vi "Calc RPM Vals.vi"(6 "RPM Loop Period (us)":u32, 10 "Sample Length(10)":u16, 11 "Inputs":bool[](array[boolean])=[FALSE, FALSE, FALSE, FALSE]) -> (3 "RPM Vals":sgl[](array[numeric]))   [LabVIEW 2018]
uses:
  <vilib>/rvi/Arithmetic/AddSubMult/XNode/nirviSatArithmetic.xnode
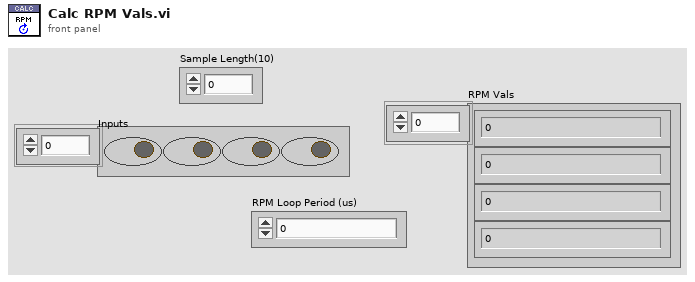
[diagram p1: front panel]
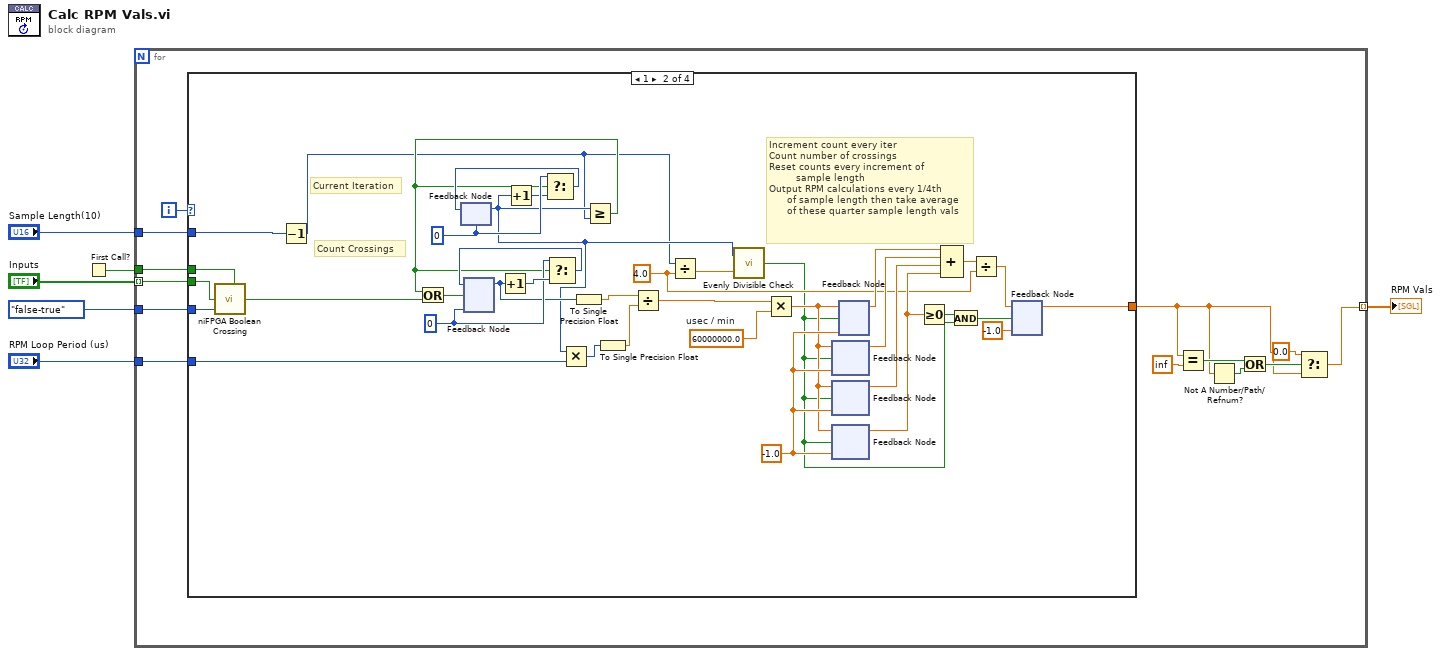
[diagram p0: block diagram]
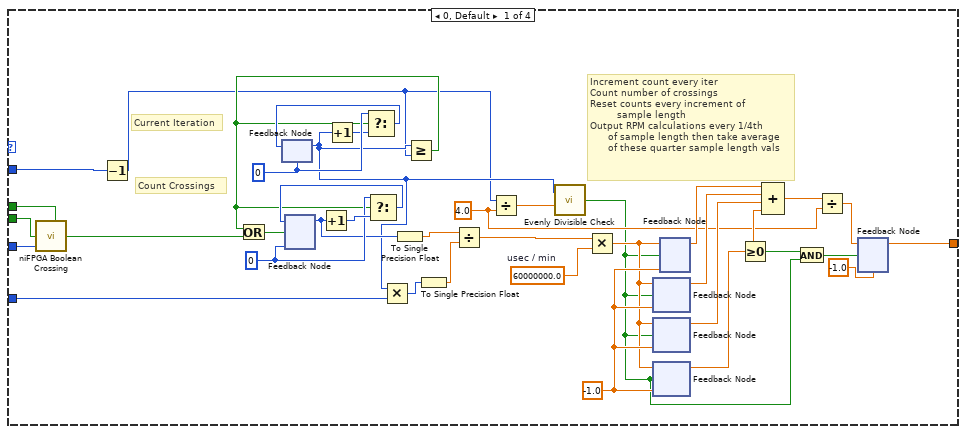
[diagram p2: hidden frame]
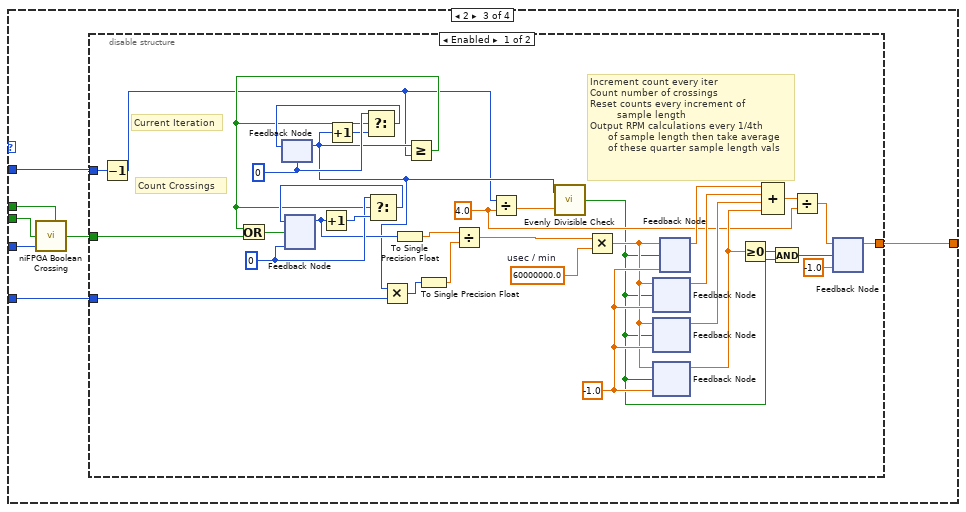
[diagram p3: hidden frame]
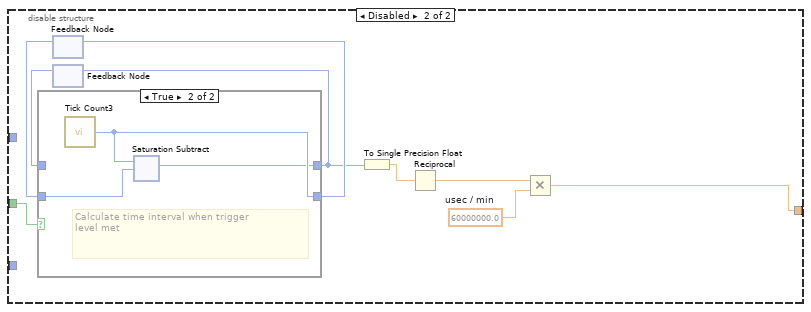
[diagram p4: hidden frame]
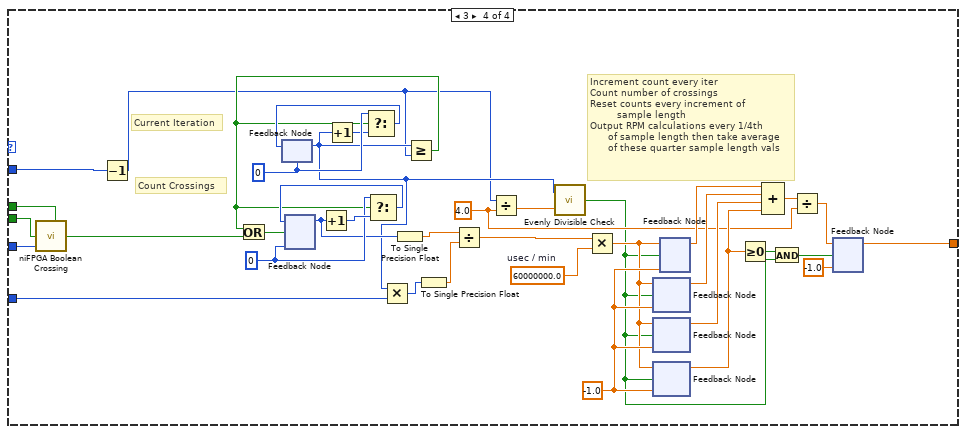
[diagram p6: hidden frame]
diagram:
  n1 = First Call?() -> (First Call?: T/F=w5:bool)
  n2 = for {
    tunnel: enum8{"either", "false-true", "true-false"}."false-true" ("direction") -> [w19]
    tunnel: w5 -> [w18]
    tunnel: "Inputs" -> [w16] mode=indexing
    tunnel: "Sample Length(10)" -> [w15]
    tunnel: [w7] -> w3 mode=indexing
    tunnel: "RPM Loop Period (us)" -> [w14]
    i -> [w17]
    n3 = case shown="1" w17 {
      tunnel: w19 -> [w56 w93 w100 w195]
      tunnel: w18 -> [w51 w88 w95 w190]
      tunnel: w16 -> [w55 w92 w99 w194]
      tunnel: w15 -> [w50 w87 w94 w189]
      tunnel: [w53 w90 w97 w192] -> w8
      tunnel: w14 -> [w52 w89 w96 w191]
      frame 0, Default {
        w25 = sgl 4.0 ("y")
        w26 = sgl -1.0
        w41 = u16 0
        w45 = u32 0
        w49 = sgl 60000000.0  # usec / min
        # "Increment count every iter\nCount number of crossings\nReset counts every increment of\n         sample length\nOutput RPM calculations every 1/4th\n      of sample length then take average\n      of these quarter sample length vals"
        # "Current Iteration"
        # "Count Crossings"
        n4 = call <vilib>:"niFPGA Boolean Crossing.vi"("input"=w55, "direction"=w56, "initialize"=w51) -> ("crossing"=w54:bool)  [unwired: 6 in]
        n5 = Decrement(x=w50) -> (x-1=w20:u16)
        n6 = feedback #1(w41) -> (w23:u16)
        n7 = feedback #2(w45) -> (w38:u32)
        n8 = Increment(x=w38) -> (x+1=w46:u32)
        n9 = Increment(x=w23) -> (x+1=w39:u16)
        n10 = Multiply(x=w23, y=w52) -> (x*y=w28:u32)
        n11 = To Single Precision Float(number=w38) -> (single precision float=w44:sgl)
        n12 = Greater Or Equal?(x=w23, y=w20) -> (x >= y?=w37:bool)
        n13 = Or(x=w37, y=w54) -> (x .or. y?=w48:bool)
        n14 = Select(t=w41, s=w37, f=w39) -> (s? t:f=w40:u16)
        n15 = feedback-in #1(w40) -> ()
        n16 = Select(t=w45, s=w37, f=w46) -> (s? t:f=w47:u32)
        n17 = feedback-in #2(w47, w48) -> ()
        n18 = To Single Precision Float(number=w28) -> (single precision float=w43:sgl)
        n19 = Divide(x=w44, y=w43) -> (x/y=w42:sgl)
        n20 = Divide(x=w20, y=w25) -> (x/y=w22:sgl)
        n21 = call "Evenly Divisible Check.vi"("y"=w22, "x"=w23) -> ("Evenly Divisible?"=w21:bool)
        n22 = Multiply(x=w42, y=w49) -> (x*y=w24:sgl)
        n23 = feedback #3(w26) -> (w34:sgl)
        n24 = feedback-in #3(w24, w21) -> ()
        n25 = feedback #4(w26) -> (w33:sgl)
        n26 = feedback-in #4(w24, w21) -> ()
        n27 = feedback #5(w26) -> (w29:sgl)
        n28 = feedback-in #5(w24, w21) -> ()
        n29 = feedback #6(w26) -> (w35:sgl)
        n30 = feedback-in #6(w24, w21) -> ()
        n31 = Greater Or Equal To 0?(x=w29) -> (x >= 0?=w30:bool)
        n32 = Compound Arithmetic op=ADD(w35, w34, w33, w29) -> (w36:sgl)
        n33 = And(x=w30, y=w21) -> (x .and. y?=w31:bool)
        n34 = Divide(x=w36, y=w25) -> (x/y=w32:sgl)
        n35 = feedback #7(sgl -1.0) -> (w53:sgl)
        n36 = feedback-in #7(w32, w31) -> ()
      }
      frame 1 {
        w62 = sgl 4.0 ("y")
        w63 = sgl -1.0
        w78 = u16 0
        w82 = u32 0
        w86 = sgl 60000000.0  # usec / min
        # "Increment count every iter\nCount number of crossings\nReset counts every increment of\n         sample length\nOutput RPM calculations every 1/4th\n      of sample length then take average\n      of these quarter sample length vals"
        # "Current Iteration"
        # "Count Crossings"
        n37 = call <vilib>:"niFPGA Boolean Crossing.vi"("input"=w92, "direction"=w93, "initialize"=w88) -> ("crossing"=w91:bool)  [unwired: 6 in]
        n38 = Decrement(x=w87) -> (x-1=w57:u16)
        n39 = feedback #8(w78) -> (w60:u16)
        n40 = feedback #9(w82) -> (w75:u32)
        n41 = Increment(x=w75) -> (x+1=w83:u32)
        n42 = Increment(x=w60) -> (x+1=w76:u16)
        n43 = Multiply(x=w60, y=w89) -> (x*y=w65:u32)
        n44 = To Single Precision Float(number=w75) -> (single precision float=w81:sgl)
        n45 = Greater Or Equal?(x=w60, y=w57) -> (x >= y?=w74:bool)
        n46 = Or(x=w74, y=w91) -> (x .or. y?=w85:bool)
        n47 = Select(t=w78, s=w74, f=w76) -> (s? t:f=w77:u16)
        n48 = feedback-in #8(w77) -> ()
        n49 = Select(t=w82, s=w74, f=w83) -> (s? t:f=w84:u32)
        n50 = feedback-in #9(w84, w85) -> ()
        n51 = To Single Precision Float(number=w65) -> (single precision float=w80:sgl)
        n52 = Divide(x=w81, y=w80) -> (x/y=w79:sgl)
        n53 = Divide(x=w57, y=w62) -> (x/y=w59:sgl)
        n54 = call "Evenly Divisible Check.vi"("y"=w59, "x"=w60) -> ("Evenly Divisible?"=w58:bool)
        n55 = Multiply(x=w79, y=w86) -> (x*y=w61:sgl)
        n56 = feedback #10(w63) -> (w71:sgl)
        n57 = feedback-in #10(w61, w58) -> ()
        n58 = feedback #11(w63) -> (w70:sgl)
        n59 = feedback-in #11(w61, w58) -> ()
        n60 = feedback #12(w63) -> (w66:sgl)
        n61 = feedback-in #12(w61, w58) -> ()
        n62 = feedback #13(w63) -> (w72:sgl)
        n63 = feedback-in #13(w61, w58) -> ()
        n64 = Greater Or Equal To 0?(x=w66) -> (x >= 0?=w67:bool)
        n65 = Compound Arithmetic op=ADD(w72, w71, w70, w66) -> (w73:sgl)
        n66 = And(x=w67, y=w58) -> (x .and. y?=w68:bool)
        n67 = Divide(x=w73, y=w62) -> (x/y=w69:sgl)
        n68 = feedback #14(sgl -1.0) -> (w90:sgl)
        n69 = feedback-in #14(w69, w68) -> ()
      }
      frame 2 {
        n70 = call <vilib>:"niFPGA Boolean Crossing.vi"("input"=w99, "direction"=w100, "initialize"=w95) -> ("crossing"=w98:bool)  [unwired: 6 in]
        n71 = disable-structure shown="Enabled" {
          disable-tunnel: w98 -> [w126 w140]
          disable-tunnel: [w116 w135] -> w97
          disable-tunnel: w96 -> [w111 _]
          disable-tunnel: w94 -> [w107 _]
          frame Enabled {
            w106 = sgl 4.0 ("y")
            w108 = sgl -1.0
            w125 = u16 0
            w130 = u32 0
            w134 = sgl 60000000.0  # usec / min
            # "Increment count every iter\nCount number of crossings\nReset counts every increment of\n         sample length\nOutput RPM calculations every 1/4th\n      of sample length then take average\n      of these quarter sample length vals"
            # "Current Iteration"
            # "Count Crossings"
            n72 = Decrement(x=w107) -> (x-1=w101:u16)
            n73 = feedback #15(w125) -> (w104:u16)
            n74 = feedback #16(w130) -> (w122:u32)
            n75 = Increment(x=w122) -> (x+1=w131:u32)
            n76 = Increment(x=w104) -> (x+1=w123:u16)
            n77 = Multiply(x=w104, y=w111) -> (x*y=w110:u32)
            n78 = To Single Precision Float(number=w122) -> (single precision float=w129:sgl)
            n79 = Greater Or Equal?(x=w104, y=w101) -> (x >= y?=w121:bool)
            n80 = Or(x=w121, y=w126) -> (x .or. y?=w133:bool)
            n81 = Select(t=w125, s=w121, f=w123) -> (s? t:f=w124:u16)
            n82 = feedback-in #15(w124) -> ()
            n83 = Select(t=w130, s=w121, f=w131) -> (s? t:f=w132:u32)
            n84 = feedback-in #16(w132, w133) -> ()
            n85 = To Single Precision Float(number=w110) -> (single precision float=w128:sgl)
            n86 = Divide(x=w129, y=w128) -> (x/y=w127:sgl)
            n87 = Divide(x=w101, y=w106) -> (x/y=w103:sgl)
            n88 = call "Evenly Divisible Check.vi"("y"=w103, "x"=w104) -> ("Evenly Divisible?"=w102:bool)
            n89 = Multiply(x=w127, y=w134) -> (x*y=w105:sgl)
            n90 = feedback #17(w108) -> (w118:sgl)
            n91 = feedback-in #17(w105, w102) -> ()
            n92 = feedback #18(w108) -> (w117:sgl)
            n93 = feedback-in #18(w105, w102) -> ()
            n94 = feedback #19(w108) -> (w112:sgl)
            n95 = feedback-in #19(w105, w102) -> ()
            n96 = feedback #20(w108) -> (w119:sgl)
            n97 = feedback-in #20(w105, w102) -> ()
            n98 = Greater Or Equal To 0?(x=w112) -> (x >= 0?=w113:bool)
            n99 = Compound Arithmetic op=ADD(w119, w118, w117, w112) -> (w120:sgl)
            n100 = And(x=w113, y=w102) -> (x .and. y?=w114:bool)
            n101 = Divide(x=w120, y=w106) -> (x/y=w115:sgl)
            n102 = feedback #21(sgl -1.0) -> (w116:sgl)
            n103 = feedback-in #21(w115, w114) -> ()
          }
          frame Disabled {
            w138 = sgl 60000000.0  # usec / min
            n104 = feedback #22() -> (w142:u32)  [unwired: 1 in]
            n105 = feedback #23() -> (w143:u32)  [unwired: 1 in]
            n106 = case shown="True" w140 {
              tunnel: w142 -> [w145 w147]
              tunnel: [w145 w148] -> w141
              tunnel: [w144 w146] -> w137
              tunnel: w143 -> [w144 _]
              frame False {
              }
              frame True {
                # "Calculate time interval when trigger\nlevel met"
                n107 = call "Tick Count3"() -> ("Tick Count(uSec)"=w148:u32)
                n108 = xnode ("Saturation Subtract")("x"=w148, "y"=w147) -> ("x-y"=w146:u32)
              }
            }
            n109 = feedback-in #22(w141) -> ()
            n110 = feedback-in #23(w137) -> ()
            n111 = To Single Precision Float(number=w137) -> (single precision float=w136:sgl)
            n112 = Reciprocal(x=w136) -> (1/x=w139:sgl)
            n113 = Multiply(x=w139, y=w138) -> (x*y=w135:sgl)
          }
        }
      }
      frame 3 {
        w164 = sgl 4.0 ("y")
        w165 = sgl -1.0
        w180 = u16 0
        w184 = u32 0
        w188 = sgl 60000000.0  # usec / min
        # "Increment count every iter\nCount number of crossings\nReset counts every increment of\n         sample length\nOutput RPM calculations every 1/4th\n      of sample length then take average\n      of these quarter sample length vals"
        # "Current Iteration"
        # "Count Crossings"
        n114 = call <vilib>:"niFPGA Boolean Crossing.vi"("input"=w194, "direction"=w195, "initialize"=w190) -> ("crossing"=w193:bool)  [unwired: 6 in]
        n115 = Decrement(x=w189) -> (x-1=w159:u16)
        n116 = feedback #24(w180) -> (w162:u16)
        n117 = feedback #25(w184) -> (w177:u32)
        n118 = Increment(x=w177) -> (x+1=w185:u32)
        n119 = Increment(x=w162) -> (x+1=w178:u16)
        n120 = Multiply(x=w162, y=w191) -> (x*y=w167:u32)
        n121 = To Single Precision Float(number=w177) -> (single precision float=w183:sgl)
        n122 = Greater Or Equal?(x=w162, y=w159) -> (x >= y?=w176:bool)
        n123 = Or(x=w176, y=w193) -> (x .or. y?=w187:bool)
        n124 = Select(t=w180, s=w176, f=w178) -> (s? t:f=w179:u16)
        n125 = feedback-in #24(w179) -> ()
        n126 = Select(t=w184, s=w176, f=w185) -> (s? t:f=w186:u32)
        n127 = feedback-in #25(w186, w187) -> ()
        n128 = To Single Precision Float(number=w167) -> (single precision float=w182:sgl)
        n129 = Divide(x=w183, y=w182) -> (x/y=w181:sgl)
        n130 = Divide(x=w159, y=w164) -> (x/y=w161:sgl)
        n131 = call "Evenly Divisible Check.vi"("y"=w161, "x"=w162) -> ("Evenly Divisible?"=w160:bool)
        n132 = Multiply(x=w181, y=w188) -> (x*y=w163:sgl)
        n133 = feedback #26(w165) -> (w173:sgl)
        n134 = feedback-in #26(w163, w160) -> ()
        n135 = feedback #27(w165) -> (w172:sgl)
        n136 = feedback-in #27(w163, w160) -> ()
        n137 = feedback #28(w165) -> (w168:sgl)
        n138 = feedback-in #28(w163, w160) -> ()
        n139 = feedback #29(w165) -> (w174:sgl)
        n140 = feedback-in #29(w163, w160) -> ()
        n141 = Greater Or Equal To 0?(x=w168) -> (x >= 0?=w169:bool)
        n142 = Compound Arithmetic op=ADD(w174, w173, w172, w168) -> (w175:sgl)
        n143 = And(x=w169, y=w160) -> (x .and. y?=w170:bool)
        n144 = Divide(x=w175, y=w164) -> (x/y=w171:sgl)
        n145 = feedback #30(sgl -1.0) -> (w192:sgl)
        n146 = feedback-in #30(w171, w170) -> ()
      }
    }
    n147 = Equal?(x=w8, y=sgl inf) -> (x = y?=w12:bool)
    n148 = Not A Number/Path/Refnum?(number/path/refnum=w8) -> (NaN/Path/Refnum?=w11:bool)
    n149 = Or(x=w12, y=w11) -> (x .or. y?=w10:bool)
    n150 = Select(t=sgl 0.0, s=w10, f=w8) -> (s? t:f=w7:sgl)
  }
  "RPM Vals" <- w3
